vi "OnResume.vi"(8 "error in (no error)":errorcluster, 11 "SnakeGame in":refnum<class "SnakeGame.lvclass">) -> (0 "error out":errorcluster, 3 "SnakeGame out":refnum<class "SnakeGame.lvclass">)   [LabVIEW 2019, in "RT_Game.lvlib" / "SnakeGame.lvclass"]
uses:
  SnakeGame.lvclass
  C:/Users/FreshBob/Dropbox/VIs/myRIO_GameConsole/RT/RT_Game/Game/Game.lvclass
  Menu/States.ctl
  Game/Game.lvclass/Game.ctl
  SnakeGame.lvclass/SnakeGame.ctl
  Game/Read Singleplayer.vi
  Game/Read SingleplayerBeforeMenu.vi
  Game/Write State.vi
  Game/Game.lvclass
  Snake/Snake.lvclass
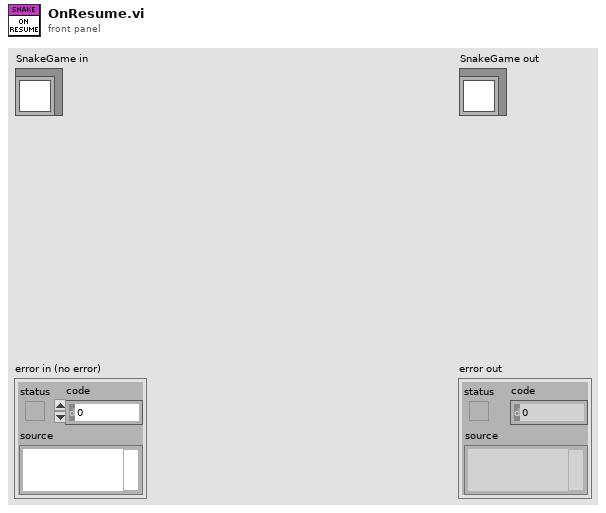
[diagram p1: front panel]
types:
  T1 = typedef "RT_Game.lvlib/Game.lvclass/States.ctl" = enum16{"Init", "Restart", "Menu", "Game", "Resume", "ToggleSingleplayer", "LoadNextGame", "ExitToMenu", "SlideOut"}
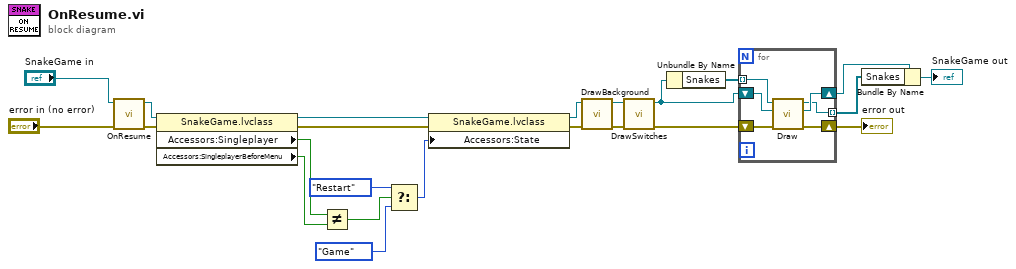
[diagram p0: block diagram]
diagram:
  n1 = call-parent "OnResume.vi"("error in (no error)"="error in (no error)", "Game in"="SnakeGame in") -> ("error out"=w15:errorcluster, "Game out"=w14:refnum<class "SnakeGame.lvclass">)  [unwired: 8 in]
  n2 = property class="SnakeGame.lvclass"(reference=w14, error in=w15) -> (reference out=w13:refnum<class "SnakeGame.lvclass">, error out=w12:errorcluster, "Accessors:Singleplayer"=w16:bool, "Accessors:SingleplayerBeforeMenu"=w17:bool)
  n3 = Not Equal?(x=w16, y=w17) -> (x != y?=w20:bool)
  n4 = Select(t=States."Restart", s=w20, f=States."Game" ("State")) -> (s? t:f=w11:T1)
  n5 = property class="SnakeGame.lvclass"(reference=w13, error in=w12, "Accessors:State"=w11) -> (reference out=w9:refnum<class "SnakeGame.lvclass">, error out=w21:errorcluster)
  n6 = call "DrawBackground.vi"("error in (no error)"=w21, "Snake in"=w9) -> ("error out"=w10:errorcluster, "Snake out"=w7:refnum<class "SnakeGame.lvclass">)  [unwired: 8 in]
  n7 = call "DrawSwitches.vi"("error in (no error)"=w10, "SnakeGame in"=w7) -> ("error out"=w8:errorcluster, "SnakeGame out"=w4:refnum<class "SnakeGame.lvclass">)  [unwired: 8 in]
  n8 = Unbundle By Name(w4) -> ("Snakes"=w3:refnum<class "Snake.lvclass">[])
  n9 = for {
    shift-right: [w28] -> w6
    shift-left: w8 -> [w29]
    shift-right: [w26] -> w5
    shift-left: w4 -> [w27]
    tunnel: w3 -> [w25] mode=indexing
    tunnel: [w24] -> w1 mode=indexing
    n10 = call "Draw.vi"("error in (no error)"=w29, "Snake in 2"=w27, "Snake in"=w25) -> ("error out"=w28:errorcluster, "Snake out 2"=w26:refnum<class "SnakeGame.lvclass">, "Snake out"=w24:refnum<class "Snake.lvclass">)  [unwired: 6 in]
  }
  "error out" <- w6
  n11 = Bundle By Name(cluster=w5, "Snakes"=w1) -> (→"SnakeGame out":refnum<class "SnakeGame.lvclass">)
